vi "Config Logging Settings.vi"(0 "VISA resource name":refnum<visa-resource-name>, 1 "Period (1)":dbl[unit]=1.0 min=1.0 max=3600.0 step=1.0, 5 "Mode (0:Off)":u16(ring) items=["Off", "Log Continuous", "Log Event", "Print Continuous", "Print Event"], 7 "Overwrite Data(F:Don't)":bool, 9 "Start (0:Clear)":u16(ring) items=["Clear", "Continuous"], 11 "error in (no error)":errorcluster, 12 "Number of Readings (1)":dbl=1.0 min=1.0 max=8.0 step=1.0) -> (4 "VISA resource name out":refnum<visa-resource-name>, 15 "error out":errorcluster)   [LabVIEW 2017, in "Lake Shore Cryotronics 218.lvlib"]
doc: "This VI configures logging parameters that apply to all readings stored. To configure individual readings use the Config. Log Readings.vi."
uses:
  Lake Shore Cryotronics 218.lvlib
panel:
  # "Overwrite\nDon't Overwrite"
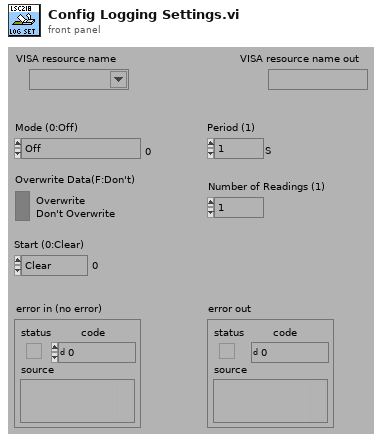
[diagram p1: front panel]
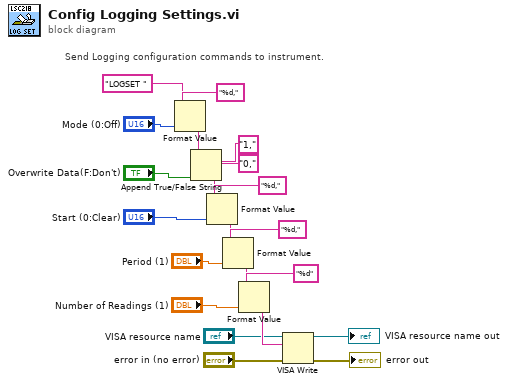
[diagram p0: block diagram]
diagram:
  # "Send Logging configuration commands to instrument."
  n1 = Format Value(string ("")="LOGSET ", format string="%d,", value (0)="Mode (0:Off)") -> (output string=w15:string)
  n2 = Append True/False String(1:"Overwrite Data(F:Don't)", 2:"0,", 3:"1,", 4:w15) -> (0:w13:string)
  n3 = Format Value(string ("")=w13, format string="%d,", value (0)="Start (0:Clear)") -> (output string=w9:string)
  n4 = Format Value(string ("")=w9, format string="%d,", value (0)="Period (1)") -> (output string=w8:string)
  n5 = Format Value(string ("")=w8, format string="%d", value (0)="Number of Readings (1)") -> (output string=w5:string)
  n6 = VISA Write(VISA resource name="VISA resource name", write buffer=w5, error in (no error)="error in (no error)") -> (VISA resource name out=→"VISA resource name out":refnum<visa-resource-name>, error out=→"error out":errorcluster)  [unwired: 1 out]
